vi "PostBuild.vi"(8 "error in (no error)":errorcluster, 9 "GeneratedFiles in":path[](array[path]), 10 "GeneratedDirectories in":path[](array[path]), 11 "Build in":refnum<class "AB_Application.lvclass">) -> (0 "error out":errorcluster, 1 "GeneratedFiles out":path[](array[path]), 2 "GeneratedDirectories out":path[](array[path]), 3 "Build out":refnum<class "AB_Application.lvclass">)   [LabVIEW 2020, in "AB_Application.lvclass"]
uses:
  <vilib>/AppBuilder/AB_Classes/Application/AB_Application.lvclass
  e:/builds/penguin/labview/branches/2020/dev/dist/vi.lib/AppBuilder/AB_Classes/Build/AB_Build.lvclass
  e:/builds/penguin/labview/branches/2020/dev/dist/vi.lib/AppBuilder/AB_Classes/TargetFile/AB_Targetfile.lvclass
  <vilib>/AppBuilder/AB_Classes/Application/AB_Application.lvclass/AB_Application.ctl
  <vilib>/AppBuilder/AB_Classes/TargetFile/AB_Targetfile.lvclass
  <vilib>/AppBuilder/CodeSignAPI/CodeSignAPI.lvlib
  <vilib>/AppBuilder/AB_Classes/Build/AB_Build.lvclass
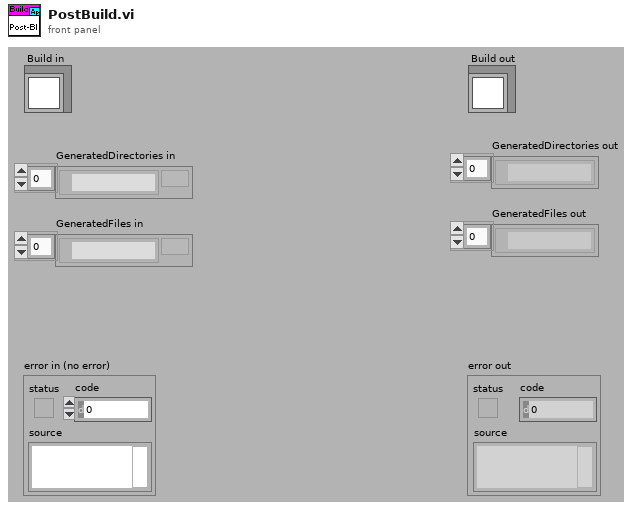
[diagram p1: front panel]
types:
  T1 = typedef "AB_Build.ctl" = cluster{"buildSpecName":string, "buildSpecDescription":string, "destinations":refnum<class "AB_Destination.lvclass">[], "exclusionOption":T2, "defaultLanguage":string, "supportedLanguages":string[], "excludedDirectories":path[], "buildContext":refnum<vi>, "buildObject":T3, "preview":bool, "programatic":bool, "progressBarEvents":T4, "userLog_Path":path, "preActionID":string, "preAction_Path":path, "postActionID":string, "postAction_Path":path, "eng_checkForBrokenVIs?":bool, "eng_verboseLinkerErrors?":bool, "localDest_Path":path, "targetDest_Path":path, "removeVIObject":u16, "cache":refnum<class "PreviewCache.lvclass">, "use cache":bool, "previewCache_ID":string, "buildCache_ID":string, "eng_TempLocalDest_Path":path, "eng_collectDependencies?":bool, "versionInfo":cluster{"buildVersion":cluster{"major":u16, "minor":u16, "patch":u16, "build":u16}, "autoIncrement":bool}, "eng_enableVIChecksums":bool}
  T2 = typedef "AB_Exclusion_Option.ctl" = cluster{"typedefs":bool, "polymorphicVIs":bool, "unusedLibraryItems":bool, "modifyLibraryFile":bool, "edit-timeDependencies":bool, "inlineVIs":bool, "dependent PPLs":bool, "dependent DLLs":bool}
  T3 = typedef "ItemRef.ctl" = u64
  T4 = typedef "provcom_ProgressBar_Events.ctl" = cluster{"newJob":refnum<user-event>, "newItem":refnum<user-event>, "errorMsg":T5, "cancel":refnum<user-event>}
  T5 = typedef "mxLvBuildError.ctl" = refnum<user-event>
  T6 = typedef "AB_Targetfile.ctl" = cluster{"targetfileName":string, "targetfileGUID":string, "enableDebugging":bool, "versionInfo":cluster{"productName":string, "legalCopyright":string, "companyName":string, "internalName":string, "fileDescription":string}, "eng_consolidatedTypeInfo":string, "fastFileFormat":bool, "eng_LEIFBuildData":u32, "versionIndependent":bool}
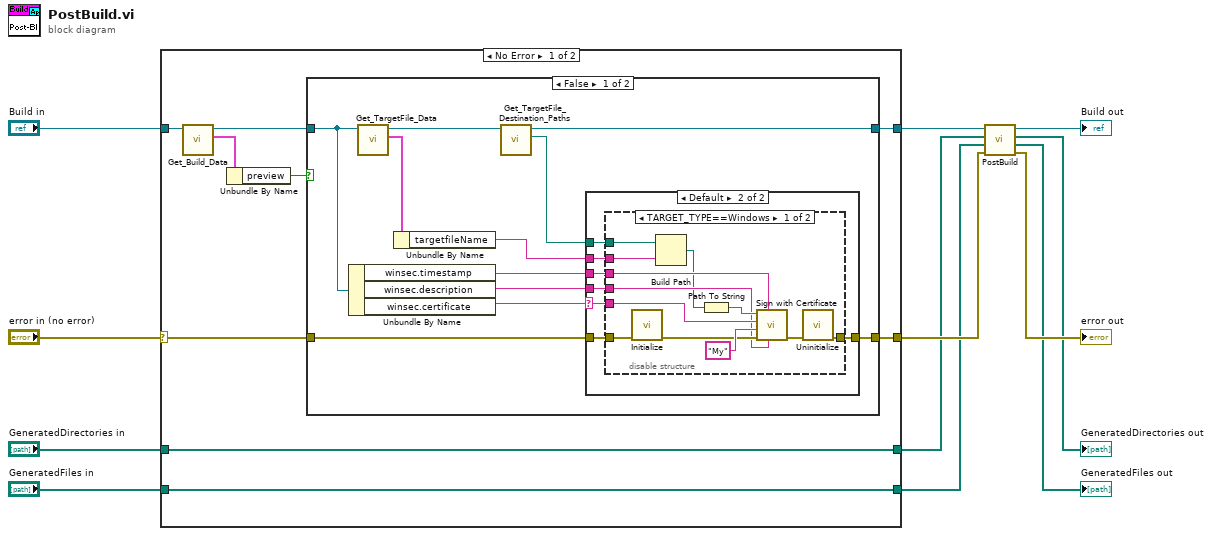
[diagram p0: block diagram]
diagram:
  n1 = case shown="No Error" "error in (no error)" {
    selector: "error in (no error)" -> [w18 w59]
    tunnel: [w17 w59] -> w5
    tunnel: [w19 w56] -> w7
    tunnel: "GeneratedFiles in" -> [w20 w58]
    tunnel: "GeneratedDirectories in" -> [w21 w57]
    tunnel: "Build in" -> [w14 w56]
    tunnel: [w21 w57] -> w4
    tunnel: [w20 w58] -> w3
    frame No Error {
      n2 = call <vilib>:"Get_Build_Data.vi"("Class in"=w14) -> ("data"=w16:T1, "Class out"=w13:refnum<class "AB_Application.lvclass">)  [unwired: 1 in, 8 out]
      n3 = Unbundle By Name(w16) -> ("preview"=w15:bool)
      n4 = case shown="False" w15 {
        tunnel: w13 -> [w25 w54]
        tunnel: [w27 w54] -> w19
        tunnel: w18 -> [w31 w55]
        tunnel: [w30 w55] -> w17
        frame False {
          n5 = Unbundle By Name(w25) -> ("winsec.timestamp"=w32:string, "winsec.description"=w29:string, "winsec.certificate"=w26:string)
          n6 = call <vilib>:"Get_TargetFile_Data.vi"("AB_Targetfile in"=w25) -> ("data"=w23:T6, "AB_Targetfile out"=w24:refnum<class "AB_Application.lvclass">)  [unwired: 8 in, 1 out]
          n7 = Unbundle By Name(w23) -> ("targetfileName"=w22:string)
          n8 = call <vilib>:"Get_TargetFile_Destination_Paths.vi"("AB_Targetfile in"=w24) -> ("destination path"=w28:path, "AB_Targetfile out"=w27:refnum<class "AB_Application.lvclass">)  [unwired: 1 in, 8 out]
          n9 = case shown="Default" w26 {
            selector: w26 -> [_ w34]
            tunnel: w32 -> [_ w40]
            tunnel: w31 -> [w33 w39]
            tunnel: [w33 w38] -> w30
            tunnel: w29 -> [_ w37]
            tunnel: w28 -> [_ w36]
            tunnel: w22 -> [_ w35]
            frame "" {
              # "Do not sign if certificate is empty"
            }
            frame Default {
              n10 = disable-structure shown="TARGET_TYPE==Windows" {
                disable-tunnel: w40 -> [w48 _]
                disable-tunnel: w39 -> [w47 w53]
                disable-tunnel: [w46 w53] -> w38
                disable-tunnel: w34 -> [w45 _]
                disable-tunnel: w37 -> [w44 _]
                disable-tunnel: w36 -> [w43 _]
                disable-tunnel: w35 -> [w41 _]
                frame condition #0 (active) {
                  n11 = call <vilib>:"Initialize.vi"("error in (no error)"=w47) -> ("error out"=w49:errorcluster)  [unwired: 10 out]
                  n12 = Build Path(base path=w43, name or relative path=w41) -> (appended path=w42:path)
                  n13 = Path To String(path=w42) -> (string=w51:string)
                  n14 = call <vilib>:"Sign with Certificate.vi"("url"=w44, "tsa"=w48, "error in (no error)"=w49, "store"="My", "certname"=w45, "filepath"=w51) -> ("error out"=w50:errorcluster)  [unwired: 5 out]
                  n15 = call <vilib>:"Uninitialize.vi"("error in (no error)"=w50) -> ("error out"=w46:errorcluster)  [unwired: 10 out]
                }
                frame condition #1 {
                }
              }
            }
          }
        }
        frame True {
        }
      }
    }
    frame Error {
    }
  }
  n16 = call-parent "PostBuild.vi"("error in (no error)"=w5, "GeneratedFiles in"=w3, "GeneratedDirectories in"=w4, "Build in"=w7) -> ("error out"=→"error out":errorcluster, "GeneratedFiles out"=→"GeneratedFiles out":path[], "GeneratedDirectories out"=→"GeneratedDirectories out":path[], "Build out"=→"Build out":refnum<class "AB_Application.lvclass">)  [unwired: 4 in]
